vi "Climber.vi"() -> ()   [LabVIEW 2012]
uses:
  ClimberState.ctl
  <vilib>/Rock Robotics/WPI/Solenoid/WPI_SolenoidValue.ctl
  <vilib>/Rock Robotics/WPI/Relay/WPI_RelayValue.ctl
  Robot Global Data.vi
  <vilib>/Rock Robotics/WPI/Solenoid/WPI_SolenoidSetEnum.vi
  <vilib>/Rock Robotics/WPI/RobotDrive/WPI_RobotDriveGetSetRefNum.vi
panel:
  in  "Debug":bool
  in  "Step":T1
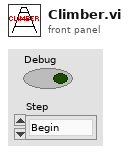
[diagram p1: front panel]
types:
  T1 = typedef "ClimberState.ctl" = enum16{"Begin", "Step 1", "Step 2", "Step 3", "Step 4", "Step 5", "Step 6", "Step 7", "Step 8", "Step 9", "Step 10", "Step 11", "Step 12", "Step 13", "Step 14", "Step 15", "Step 16", "Step 17", "Step 18", "Step 19", "Step 20", "Step 21", "Step 22", "Step 23", "End"}
  T2 = typedef "WPI_SolenoidValue.ctl" = enum16{"Off", "On", "Forward", "Reverse"}
  T3 = typedef "WPI_RelayValue.ctl" = enum16{"Off", "On", "Forward", "Reverse"}
  T4 = typedef "Level state.ctl" = enum16{"None", "Level 1", "Level 2", "Level 3"}
  T5 = typedef "WPI_SolenoidDevRef.ctl" = cluster{"DevStatus":errorcluster, "Solenoid Module":T6, "Forward Solenoid Channel":T7, "Reverse Solenoid Channel":T7}
  T6 = typedef "FPGA_TypedefSolenoidModule.ctl" = enum16{"Solenoid Module 1", "Solenoid Module 2"}
  T7 = typedef "WPI_SolenoidChannel.ctl" = enum8{"Solenoid 1", "Solenoid 2", "Solenoid 3", "Solenoid 4", "Solenoid 5", "Solenoid 6", "Solenoid 7", "Solenoid 8", "Invalid"}
  T8 = typedef "WPI_MotorControlDeviceRef.ctl" = cluster{"DeviceStatus":errorcluster, "Type":enum16{"PWM", "CAN"}, "PWM":cluster{"Digital Module":T9, "PWM Channel":T10, "DeadBand":T11}, "CAN":cluster{"Device Number":u8, "Control Mode":T12, "Semaphore":T13, "Max Vout":dbl}, "Invert":bool, "TransformRef":T14, "InvTransformRef":T14}
  T9 = typedef "FPGA_TypedefDigitalModule.ctl" = enum16{"Digital Module 1", "Digital Module 2"}
  T10 = typedef "FPGA_DIOPWMChannel.ctl" = enum8{"PWM 1", "PWM 2", "PWM 3", "PWM 4", "PWM 5", "PWM 6", "PWM 7", "PWM 8", "PWM 9", "PWM 10", "Invalid"}
  T11 = typedef "WPI_PWMDeadband.ctl" = cluster{"Name":string, "maxPositivePwm":i32, "minPositivePwm":i32, "centerPwm":i32, "maxNegativePwm":i32, "minNegativePwm":i32, "angularRange":u16}
  T12 = typedef "WPI_CANJaguar_ControlMode.ctl" = enum8{"Percent VBus", "Current", "Speed", "Position", "Voltage"}
  T13 = typedef "Semaphore RefNum" = refnum<k1>
  T14 = typedef "WPI_PWMTransform_ConPane.ctl" = refnum<vi>
  T15 = typedef "WPI_RobotDriveDevRef.ctl" = cluster{"DevStatus":errorcluster, "Motors[]":T8[], "Square Inputs":bool, "Max Output":dbl, "Isochronous":bool}
  T16 = typedef "WPI_RelayDevRef.ctl" = cluster{"DevStatus":errorcluster, "Relay Channel":T17, "Digital Module":T9, "Relay Direction":T18}
  T17 = typedef "FPGA_DIORelayChannel.ctl" = enum8{"Relay 1", "Relay 2", "Relay 3", "Relay 4", "Relay 5", "Relay 6", "Relay 7", "Relay 8", "Invalid"}
  T18 = typedef "WPI_RelayDirection.ctl" = enum16{"Both directions", "Forward only", "Reverse only"}
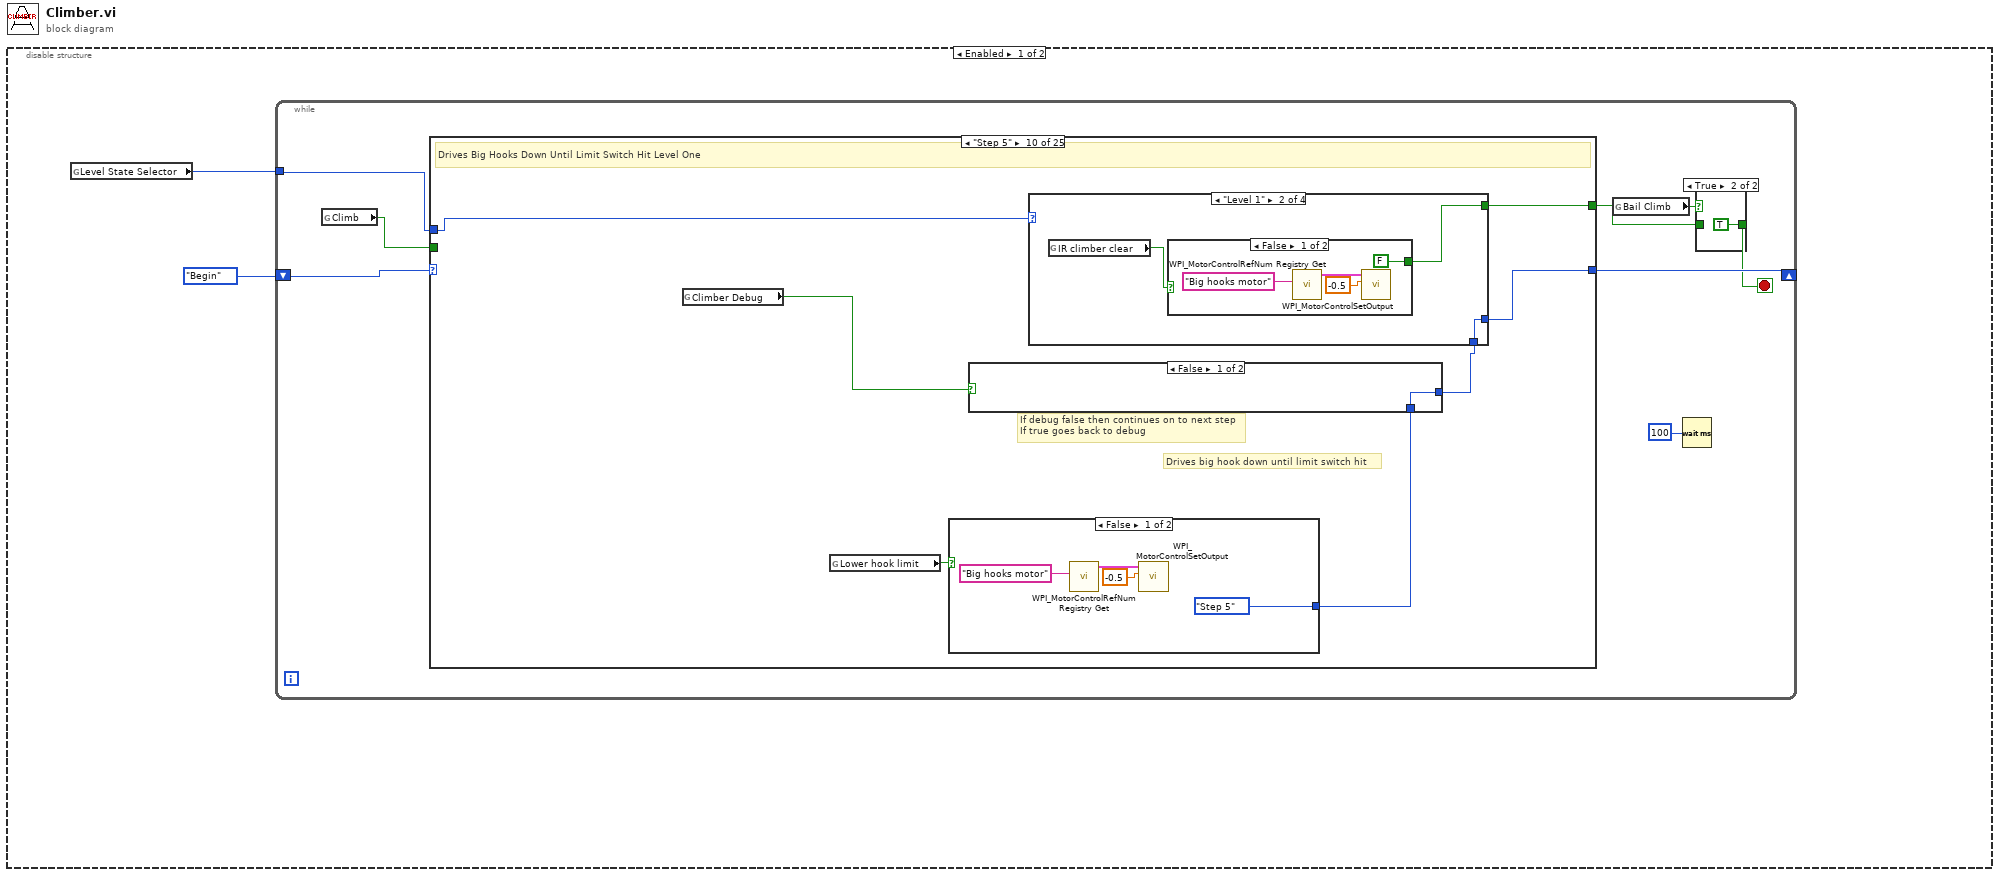
[diagram p0: block diagram]
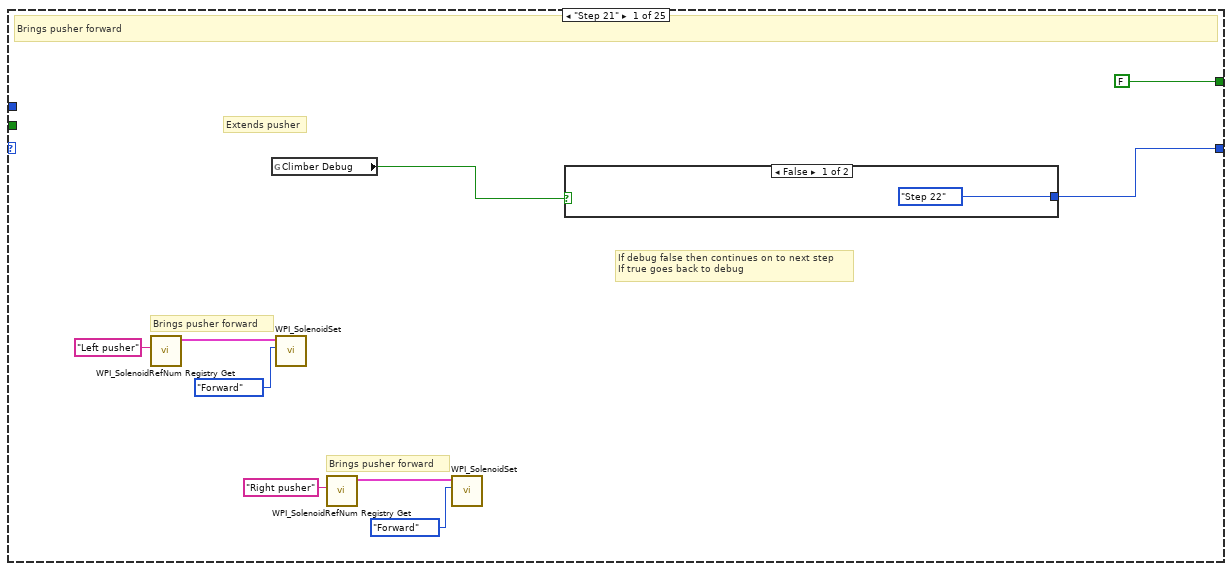
[diagram p3: hidden frame]
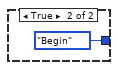
[diagram p4: hidden frame]
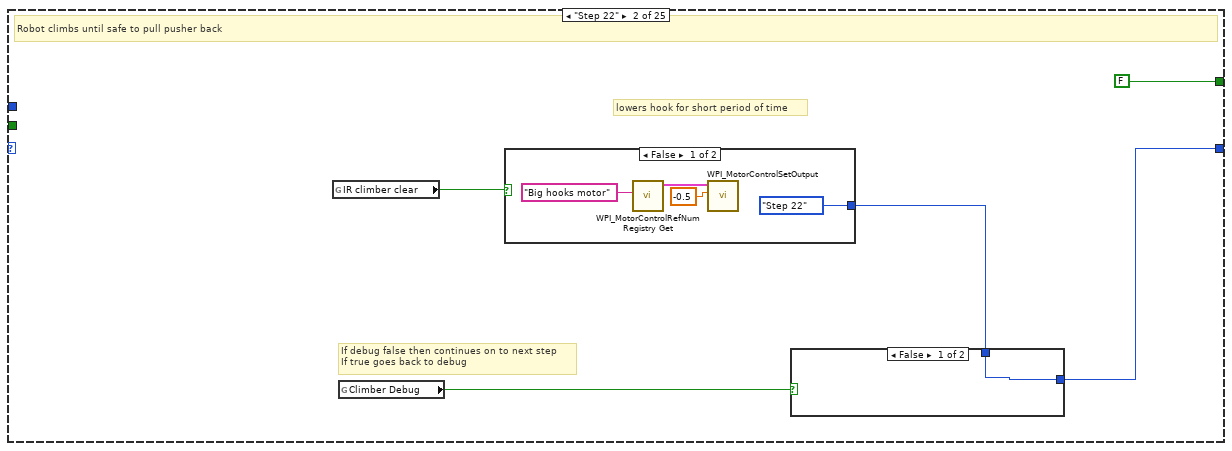
[diagram p5: hidden frame]
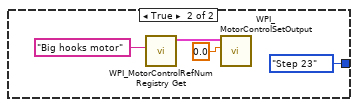
[diagram p6: hidden frame]
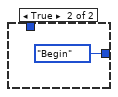
[diagram p7: hidden frame]
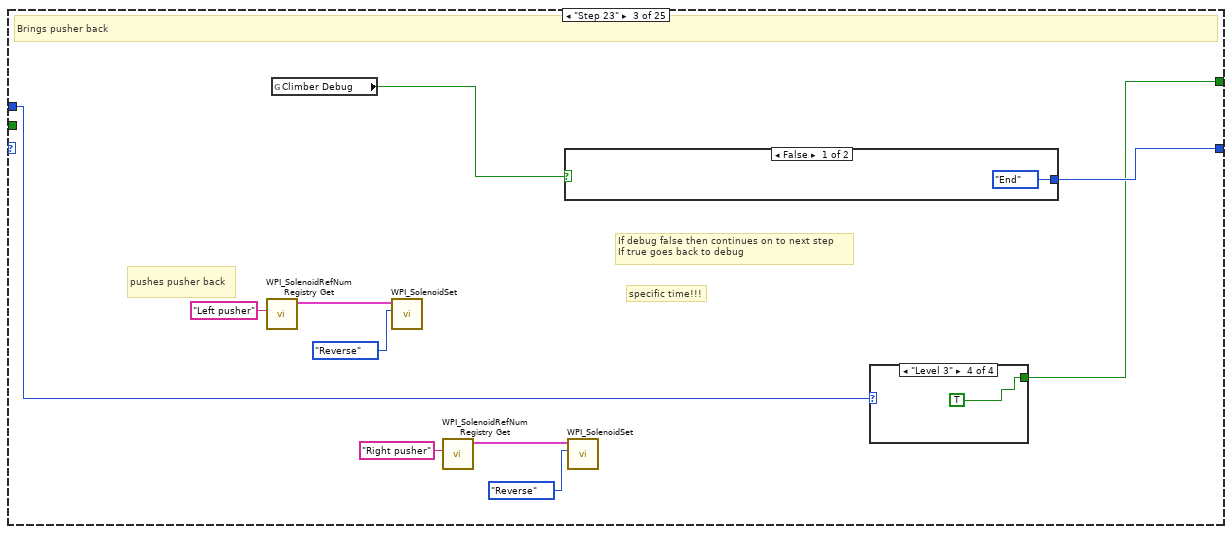
[diagram p8: hidden frame]
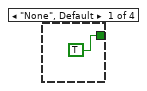
[diagram p9: hidden frame]
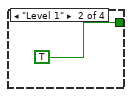
[diagram p10: hidden frame]
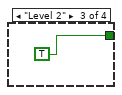
[diagram p11: hidden frame]
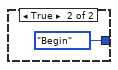
[diagram p12: hidden frame]
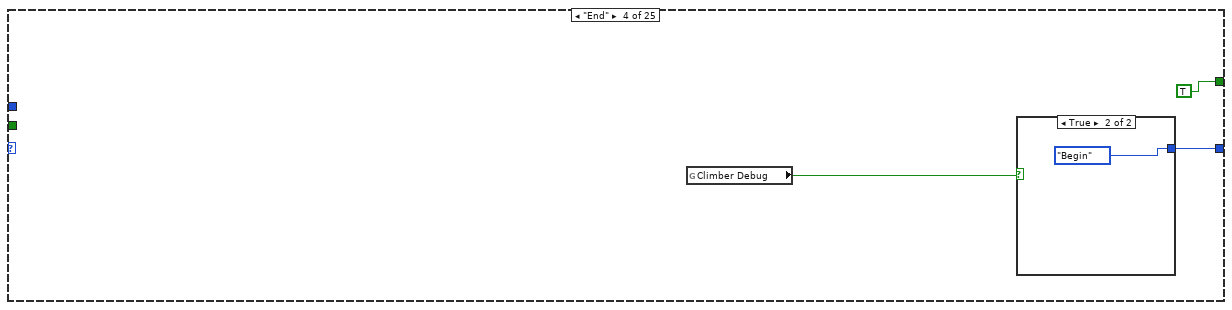
[diagram p13: hidden frame]
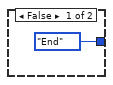
[diagram p14: hidden frame]
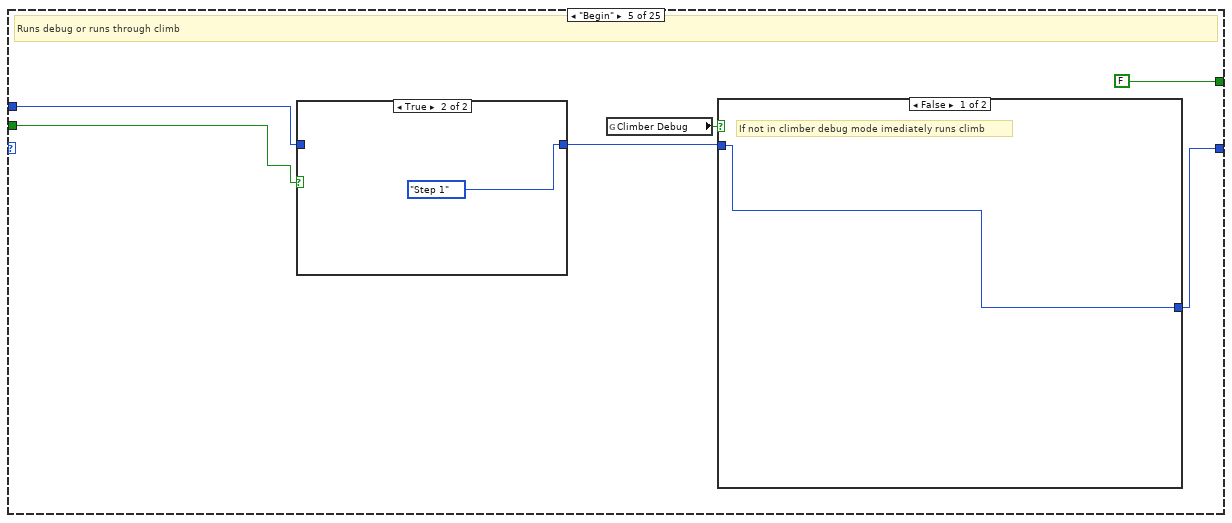
[diagram p15: hidden frame]
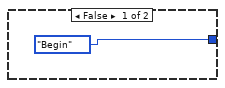
[diagram p16: hidden frame]
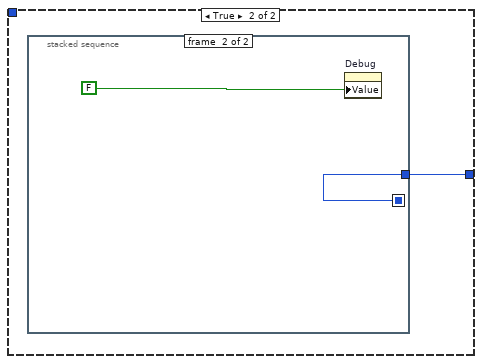
[diagram p17: hidden frame]
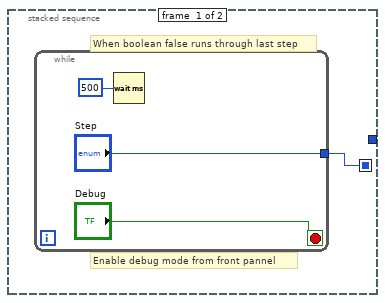
[diagram p18: hidden frame]
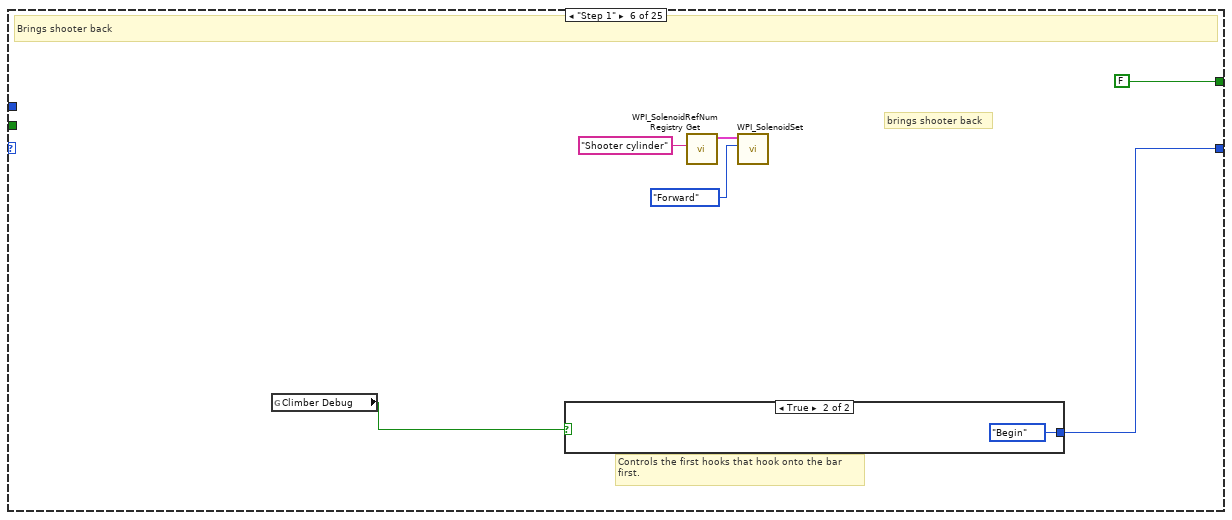
[diagram p19: hidden frame]
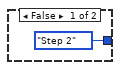
[diagram p20: hidden frame]
diagram:
  n1 = disable-structure shown="Enabled" {
    frame Enabled {
      n2 = global read "Robot Global Data.vi" "Level State Selector"() -> (w2:T4)
      n3 = while {
        shift-right: [w10] -> _
        shift-left: ClimberState."Begin" ("Enum") -> [w9]
        tunnel: w2 -> [w4]
        stop <- w8 stop-if-true
        n4 = global read "Robot Global Data.vi" "Climb"() -> (w3:bool)
        n5 = case shown="\"Step 5\"" w9 {
          tunnel: [w19 w26 w47 w56 w65 w80 w85 w104 w112 w117 w154 w160 w172 w190 w206 w217 w224 w245 w255 w271 w277 w289 w305 w312 w328] -> w10
          tunnel: [FALSE FALSE w40 TRUE FALSE FALSE FALSE FALSE FALSE w120 FALSE FALSE FALSE FALSE FALSE FALSE FALSE w238 FALSE FALSE FALSE FALSE FALSE FALSE FALSE] -> w7
          tunnel: w4 -> [_ _ w39 _ w62 _ _ _ _ w119 _ _ _ _ _ _ _ w237 _ _ _ _ _ _ _]
          tunnel: w3 -> [_ _ _ _ w60 _ _ _ _ _ _ _ _ _ _ _ _ _ _ _ _ _ _ _ _]
          frame "Step 21" {
            # "Brings pusher forward"
            # "Brings pusher forward"
            # "If debug false then continues on to next step\nIf true goes back to debug"
            # "Extends pusher"
            # "Brings pusher forward"
            n6 = call <vilib>:"WPI_SolenoidRefNum Registry Get.vi"("refnum name"="Left pusher") -> ("SolenoidDevRef"=w16:T5)  [unwired: 9 in, 1 out]
            n7 = global read "Robot Global Data.vi" "Climber Debug"() -> (w20:bool)
            n8 = call-poly <vilib>:"WPI_SolenoidSet.vi"("Value"=WPI_SolenoidValue."Forward", "SolenoidDevRef"=w16) -> ()  [unwired: 8 in, 2 out]
            n9 = call <vilib>:"WPI_SolenoidRefNum Registry Get.vi"("refnum name"="Right pusher") -> ("SolenoidDevRef"=w14:T5)  [unwired: 9 in, 1 out]
            n10 = call-poly <vilib>:"WPI_SolenoidSet.vi"("Value"=WPI_SolenoidValue."Forward", "SolenoidDevRef"=w14) -> ()  [unwired: 8 in, 2 out]
            n11 = case shown="False" w20 {
              tunnel: [ClimberState."Step 22" ("Enum") ClimberState."Begin" ("Enum")] -> w19
              frame False {
              }
              frame True {
              }
            }
          }
          frame "Step 22" {
            # "lowers hook for short period of time"
            # "If debug false then continues on to next step\nIf true goes back to debug"
            # "Robot climbs until safe to pull pusher back"
            n12 = global read "Robot Global Data.vi" "IR climber clear"() -> (w25:bool)
            n13 = global read "Robot Global Data.vi" "Climber Debug"() -> (w27:bool)
            n14 = case shown="False" w25 {
              tunnel: [ClimberState."Step 22" ("Enum") ClimberState."Step 23" ("Enum")] -> w24
              frame False {
                n15 = call <vilib>:"WPI_MotorControlRefNum Registry Get.vi"("refnum name"="Big hooks motor") -> ("MotorControlDevRef"=w30:T8)  [unwired: 9 in, 1 out]
                n16 = call <vilib>:"WPI_MotorControlSetOutput.vi"("Output"=-0.5, "MotorControlDevRef"=w30) -> ()  [unwired: 7 in, 3 out]
              }
              frame True {
                n17 = call <vilib>:"WPI_MotorControlRefNum Registry Get.vi"("refnum name"="Big hooks motor") -> ("MotorControlDevRef"=w36:T8)  [unwired: 9 in, 1 out]
                n18 = call <vilib>:"WPI_MotorControlSetOutput.vi"("Output"=0.0, "MotorControlDevRef"=w36) -> ()  [unwired: 7 in, 3 out]
              }
            }
            n19 = case shown="False" w27 {
              tunnel: [w37 ClimberState."Begin" ("Enum")] -> w26
              tunnel: w24 -> [w37 _]
              frame False {
              }
              frame True {
              }
            }
          }
          frame "Step 23" {
            # "specific time!!!"
            # "pushes pusher back"
            # "If debug false then continues on to next step\nIf true goes back to debug"
            # "Brings pusher back"
            n20 = call <vilib>:"WPI_SolenoidRefNum Registry Get.vi"("refnum name"="Left pusher") -> ("SolenoidDevRef"=w44:T5)  [unwired: 9 in, 1 out]
            n21 = global read "Robot Global Data.vi" "Climber Debug"() -> (w48:bool)
            n22 = call-poly <vilib>:"WPI_SolenoidSet.vi"("Value"=WPI_SolenoidValue."Reverse", "SolenoidDevRef"=w44) -> ()  [unwired: 8 in, 2 out]
            n23 = call <vilib>:"WPI_SolenoidRefNum Registry Get.vi"("refnum name"="Right pusher") -> ("SolenoidDevRef"=w42:T5)  [unwired: 9 in, 1 out]
            n24 = case shown="False" w48 {
              tunnel: [ClimberState."End" ("Enum") ClimberState."Begin" ("Enum")] -> w47
              frame False {
              }
              frame True {
              }
            }
            n25 = call-poly <vilib>:"WPI_SolenoidSet.vi"("Value"=WPI_SolenoidValue."Reverse", "SolenoidDevRef"=w42) -> ()  [unwired: 8 in, 2 out]
            n26 = case shown="\"Level 3\"" w39 {
              tunnel: [TRUE TRUE TRUE TRUE] -> w40
              frame "None", Default {
              }
              frame "Level 1" {
              }
              frame "Level 2" {
              }
              frame "Level 3" {
              }
            }
          }
          frame "End" {
            n27 = global read "Robot Global Data.vi" "Climber Debug"() -> (w55:bool)
            n28 = case shown="True" w55 {
              tunnel: [ClimberState."End" ("Enum") ClimberState."Begin" ("Enum")] -> w56
              frame False {
              }
              frame True {
              }
            }
          }
          frame "Begin" {
            # "Runs debug or runs through climb"
            n29 = case shown="True" w60 {
              tunnel: w62 -> [_ _]
              tunnel: [ClimberState."Begin" ("Enum") ClimberState."Step 1" ("Enum")] -> w61
              frame False {
              }
              frame True {
              }
            }
            n30 = global read "Robot Global Data.vi" "Climber Debug"() -> (w63:bool)
            n31 = case shown="False" w63 {
              tunnel: [w68 w69] -> w65
              tunnel: w61 -> [w68 _]
              frame False {
                # "If not in climber debug mode imediately runs climb"
              }
              frame True {
                n32 = stacked-sequence {
                  seq-local: [w70 _] -> [_ w75]
                  tunnel: [_ w75] -> w69
                  frame #0 {
                    # "When boolean false runs through last step"
                    # "Enable debug mode from front pannel"
                    n33 = while {
                      tunnel: ["Step"] -> w70
                      stop <- "Debug" stop-if-true
                      n34 = Wait (ms)(milliseconds to wait=u32 500) -> ()  [unwired: 1 out]
                    }
                  }
                  frame #1 {
                    n35 = property on="Debug" class="Bool (strict)"("Value"=FALSE ("Debug")) -> ()  [unwired: 2 in, 2 out]
                  }
                }
              }
            }
          }
          frame "Step 1" {
            # "brings shooter back"
            # "Controls the first hooks that hook onto the bar\nfirst."
            # "Brings shooter back"
            n36 = global read "Robot Global Data.vi" "Climber Debug"() -> (w79:bool)
            n37 = case shown="True" w79 {
              tunnel: [ClimberState."Step 2" ("Enum") ClimberState."Begin" ("Enum")] -> w80
              frame False {
              }
              frame True {
              }
            }
            n38 = call <vilib>:"WPI_SolenoidRefNum Registry Get.vi"("refnum name"="Shooter cylinder") -> ("SolenoidDevRef"=w77:T5)  [unwired: 9 in, 1 out]
            n39 = call-poly <vilib>:"WPI_SolenoidSet.vi"("Value"=WPI_SolenoidValue."Forward", "SolenoidDevRef"=w77) -> ()  [unwired: 8 in, 2 out]
          }
          frame "Step 2" {
            # "Drives hook up till limit switch hit"
            # "till hits limit switch"
            # "If debug false then continues on to next step\nIf true goes back to debug"
            # "Drives up to bar"
            # "Drives big hooks up"
            n40 = global read "Robot Global Data.vi" "Climber Debug"() -> (w87:bool)
            n41 = global read "Robot Global Data.vi" "Top hook limit"() -> (w86:bool)
            n42 = case shown="False" w86 {
              tunnel: [ClimberState."Step 2" ("Enum") ClimberState."Step 3" ("Enum")] -> w84
              frame False {
                n43 = call <vilib>:"WPI_MotorControlRefNum Registry Get.vi"("refnum name"="Big hooks motor") -> ("MotorControlDevRef"=w90:T8)  [unwired: 9 in, 1 out]
                n44 = call <vilib>:"WPI_MotorControlSetOutput.vi"("Output"=0.5, "MotorControlDevRef"=w90) -> ()  [unwired: 7 in, 3 out]
              }
              frame True {
                n45 = call <vilib>:"WPI_MotorControlRefNum Registry Get.vi"("refnum name"="Big hooks motor") -> ("MotorControlDevRef"=w96:T8)  [unwired: 9 in, 1 out]
                n46 = call <vilib>:"WPI_MotorControlSetOutput.vi"("Output"=0.0, "MotorControlDevRef"=w96) -> ()  [unwired: 7 in, 3 out]
              }
            }
            n47 = case shown="True" w87 {
              tunnel: [w97 ClimberState."Begin" ("Enum")] -> w85
              tunnel: w84 -> [w97 _]
              frame False {
              }
              frame True {
              }
            }
          }
          frame "Step 3" {
            # "Drives robot up to the tower"
            # "If debug false then continues on to next step\nIf true goes back to debug"
            # "Drives robot to tower"
            n48 = global read "Robot Global Data.vi" "Climber Debug"() -> (w105:bool)
            n49 = call <vilib>:"WPI_RobotDriveRefNum Registry Get.vi"("refnum name"="Left and Right Motors") -> ("error out"=w103:errorcluster, "RobotDriveDevRef"=w102:T15)  [unwired: 1 in, 8 out]
            n50 = call <vilib>:"WPI_RobotDriveTankDrive.vi"("error in (no error)"=w103, "Right axis value"=-0.5, "Left axis value"=-0.5, "RobotDriveDevRef"=w102) -> ()  [unwired: 5 in, 3 out]
            n51 = case shown="True" w105 {
              tunnel: [ClimberState."Step 4" ("Enum") ClimberState."Begin" ("Enum")] -> w104
              frame False {
              }
              frame True {
              }
            }
          }
          frame "Step 4" {
            # "Makes sure that Ratchet is engaged"
            # "If debug false then continues on to next step\nIf true goes back to debug"
            # "Brings Ratchet Forward to Ensure that it is Engaged"
            n52 = global read "Robot Global Data.vi" "Climber Debug"() -> (w113:bool)
            n53 = case shown="False" w113 {
              tunnel: [ClimberState."Step 5" ("Enum") ClimberState."Begin" ("Enum")] -> w112
              frame False {
              }
              frame True {
              }
            }
            n54 = call <vilib>:"WPI_SolenoidRefNum Registry Get.vi"("refnum name"="Big hooks lock") -> ("SolenoidDevRef"=w110:T5)  [unwired: 9 in, 1 out]
            n55 = call-poly <vilib>:"WPI_SolenoidSet.vi"("Value"=WPI_SolenoidValue."Forward", "SolenoidDevRef"=w110) -> ()  [unwired: 8 in, 2 out]
          }
          frame "Step 5" {
            # "Drives big hook down until limit switch hit"
            # "If debug false then continues on to next step\nIf true goes back to debug"
            # "Drives Big Hooks Down Until Limit Switch Hit Level One"
            n56 = global read "Robot Global Data.vi" "Climber Debug"() -> (w123:bool)
            n57 = global read "Robot Global Data.vi" "Lower hook limit"() -> (w122:bool)
            n58 = case shown="False" w122 {
              tunnel: [ClimberState."Step 5" ("Enum") ClimberState."Step 6" ("Enum")] -> w121
              frame False {
                n59 = call <vilib>:"WPI_MotorControlRefNum Registry Get.vi"("refnum name"="Big hooks motor") -> ("MotorControlDevRef"=w142:T8)  [unwired: 9 in, 1 out]
                n60 = call <vilib>:"WPI_MotorControlSetOutput.vi"("Output"=-0.5, "MotorControlDevRef"=w142) -> ()  [unwired: 7 in, 3 out]
              }
              frame True {
                n61 = call <vilib>:"WPI_MotorControlRefNum Registry Get.vi"("refnum name"="Big hooks motor") -> ("MotorControlDevRef"=w148:T8)  [unwired: 9 in, 1 out]
                n62 = call <vilib>:"WPI_MotorControlSetOutput.vi"("Output"=0.0, "MotorControlDevRef"=w148) -> ()  [unwired: 7 in, 3 out]
              }
            }
            n63 = case shown="False" w123 {
              tunnel: [w149 ClimberState."Begin" ("Enum")] -> w118
              tunnel: w121 -> [w149 _]
              frame False {
              }
              frame True {
              }
            }
            n64 = case shown="\"Level 1\"" w119 {
              tunnel: [TRUE w126 FALSE FALSE] -> w120
              tunnel: w118 -> [w124 w127 w137 w139]
              tunnel: [w124 w127 w137 w139] -> w117
              frame "None", Default {
              }
              frame "Level 1" {
                n65 = global read "Robot Global Data.vi" "IR climber clear"() -> (w128:bool)
                n66 = case shown="False" w128 {
                  tunnel: [FALSE TRUE] -> w126
                  frame False {
                    n67 = call <vilib>:"WPI_MotorControlRefNum Registry Get.vi"("refnum name"="Big hooks motor") -> ("MotorControlDevRef"=w132:T8)  [unwired: 9 in, 1 out]
                    n68 = call <vilib>:"WPI_MotorControlSetOutput.vi"("Output"=-0.5, "MotorControlDevRef"=w132) -> ()  [unwired: 7 in, 3 out]
                  }
                  frame True {
                    n69 = call <vilib>:"WPI_MotorControlRefNum Registry Get.vi"("refnum name"="Big hooks motor") -> ("MotorControlDevRef"=w136:T8)  [unwired: 9 in, 1 out]
                    n70 = call <vilib>:"WPI_MotorControlSetOutput.vi"("Output"=0.0, "MotorControlDevRef"=w136) -> ()  [unwired: 7 in, 3 out]
                  }
                }
              }
              frame "Level 2" {
              }
              frame "Level 3" {
              }
            }
          }
          frame "Step 6" {
            # "pushes inner hooks forward"
            # "Extends Outer Hook"
            # "If debug false then continues on to next step\nIf true goes back to debug"
            # "Brings Small Hooks Forward onto Bar"
            n71 = global read "Robot Global Data.vi" "Climber Debug"() -> (w155:bool)
            n72 = call <vilib>:"WPI_RelayRefNum Registry Get.vi"("refnum name"="Small hooks") -> ("RelayDevRef"=w153:T16)  [unwired: 9 in, 1 out]
            n73 = call <vilib>:"WPI_RelaySet.vi"("RelayValue"=WPI_RelayValue."Forward", "RelayDevRef"=w153) -> ()  [unwired: 8 in, 2 out]
            n74 = case shown="False" w155 {
              tunnel: [ClimberState."Step 7" ("Enum") ClimberState."Begin" ("Enum")] -> w154
              frame False {
              }
              frame True {
              }
            }
          }
          frame "Step 7" {
            # "Brings ratchet back then drives down for short moment"
            # "If debug false then continues on to next step\nIf true goes back to debug"
            # "Brings ratchet back and drives down"
            n75 = flat-sequence {
              frame #0 {
                n76 = call <vilib>:"WPI_SolenoidRefNum Registry Get.vi"("refnum name"="Big hooks lock") -> ("SolenoidDevRef"=w163:T5)  [unwired: 9 in, 1 out]
                n77 = call-poly <vilib>:"WPI_SolenoidSet.vi"("Value"=WPI_SolenoidValue."Reverse", "SolenoidDevRef"=w163) -> ()  [unwired: 8 in, 2 out]
              }
              frame #1 {
                n78 = call <vilib>:"WPI_MotorControlRefNum Registry Get.vi"("refnum name"="Big hooks motor") -> ("MotorControlDevRef"=w167:T8)  [unwired: 9 in, 1 out]
                n79 = call <vilib>:"WPI_MotorControlSetOutput.vi"("Output"=-0.5, "MotorControlDevRef"=w167) -> ()  [unwired: 7 in, 3 out]
              }
            }
            n80 = global read "Robot Global Data.vi" "Climber Debug"() -> (w161:bool)
            n81 = case shown="False" w161 {
              tunnel: [ClimberState."Step 8" ("Enum") ClimberState."Begin" ("Enum")] -> w160
              frame False {
              }
              frame True {
              }
            }
          }
          frame "Step 8" {
            # "till hits limit switch"
            # "If debug false then continues on to next step\nIf true goes back to debug"
            # "Extends inner hooks"
            # "Brings big hook up until limit switch hit"
            n82 = global read "Robot Global Data.vi" "Climber Debug"() -> (w173:bool)
            n83 = global read "Robot Global Data.vi" "Top hook limit"() -> (w171:bool)
            n84 = case shown="False" w171 {
              tunnel: [ClimberState."Step 8" ("Enum") ClimberState."Step 9" ("Enum")] -> w170
              frame False {
                n85 = call <vilib>:"WPI_MotorControlRefNum Registry Get.vi"("refnum name"="Big hooks motor") -> ("MotorControlDevRef"=w176:T8)  [unwired: 9 in, 1 out]
                n86 = call <vilib>:"WPI_MotorControlSetOutput.vi"("Output"=0.5, "MotorControlDevRef"=w176) -> ()  [unwired: 7 in, 3 out]
              }
              frame True {
                n87 = call <vilib>:"WPI_MotorControlRefNum Registry Get.vi"("refnum name"="Big hooks motor") -> ("MotorControlDevRef"=w182:T8)  [unwired: 9 in, 1 out]
                n88 = call <vilib>:"WPI_MotorControlSetOutput.vi"("Output"=0.0, "MotorControlDevRef"=w182) -> ()  [unwired: 7 in, 3 out]
              }
            }
            n89 = case shown="False" w173 {
              tunnel: [w183 ClimberState."Begin" ("Enum")] -> w172
              tunnel: w170 -> [w183 _]
              frame False {
              }
              frame True {
              }
            }
          }
          frame "Step 9" {
            # "Ratchet engages."
            # "If debug false then continues on to next step\nIf true goes back to debug"
            # "Brings Ratchet forward and lowers big hook"
            n90 = call <vilib>:"WPI_SolenoidRefNum Registry Get.vi"("refnum name"="Big hooks lock") -> ("SolenoidDevRef"=w188:T5)  [unwired: 9 in, 1 out]
            n91 = call-poly <vilib>:"WPI_SolenoidSet.vi"("Value"=WPI_SolenoidValue."Forward", "SolenoidDevRef"=w188) -> ()  [unwired: 8 in, 2 out]
            n92 = global read "Robot Global Data.vi" "Climber Debug"() -> (w191:bool)
            n93 = global read "Robot Global Data.vi" "Big Hooks on Bar"() -> (w186:bool)
            n94 = case shown="False" w186 {
              tunnel: [ClimberState."Step 9" ("Enum") ClimberState."Step 10" ("Enum")] -> w185
              frame False {
                # "Lowers the big hooks"
                n95 = call <vilib>:"WPI_MotorControlRefNum Registry Get.vi"("refnum name"="Big hooks motor") -> ("MotorControlDevRef"=w196:T8)  [unwired: 9 in, 1 out]
                n96 = call <vilib>:"WPI_MotorControlSetOutput.vi"("Output"=-0.5, "MotorControlDevRef"=w196) -> ()  [unwired: 7 in, 3 out]
              }
              frame True {
                n97 = call <vilib>:"WPI_MotorControlRefNum Registry Get.vi"("refnum name"="Big hooks motor") -> ("MotorControlDevRef"=w199:T8)  [unwired: 9 in, 1 out]
                n98 = call <vilib>:"WPI_MotorControlSetOutput.vi"("Output"=0.0, "MotorControlDevRef"=w199) -> ()  [unwired: 7 in, 3 out]
              }
            }
            n99 = case shown="False" w191 {
              tunnel: [w201 ClimberState."Begin" ("Enum")] -> w190
              tunnel: w185 -> [w201 _]
              frame False {
              }
              frame True {
              }
            }
          }
          frame "Step 10" {
            # "Bring small inner hooks back"
            # "If debug false then continues on to next step\nIf true goes back to debug"
            # "Brings small inner hooks back"
            n100 = global read "Robot Global Data.vi" "Climber Debug"() -> (w207:bool)
            n101 = call <vilib>:"WPI_RelayRefNum Registry Get.vi"("refnum name"="Small hooks") -> ("RelayDevRef"=w205:T16)  [unwired: 9 in, 1 out]
            n102 = case shown="False" w207 {
              tunnel: [ClimberState."Step 11" ("Enum") ClimberState."Begin" ("Enum")] -> w206
              frame False {
              }
              frame True {
              }
            }
            n103 = call <vilib>:"WPI_RelaySet.vi"("RelayValue"=WPI_RelayValue."Reverse", "RelayDevRef"=w205) -> ()  [unwired: 8 in, 2 out]
          }
          frame "Step 11" {
            # "Brings pusher forward"
            # "If debug false then continues on to next step\nIf true goes back to debug"
            # "Brings pusher forward"
            # "Extends inner hooks"
            # "Pusher pushes robot forward"
            n104 = global read "Robot Global Data.vi" "Climber Debug"() -> (w218:bool)
            n105 = call <vilib>:"WPI_SolenoidRefNum Registry Get.vi"("refnum name"="Left pusher") -> ("SolenoidDevRef"=w214:T5)  [unwired: 9 in, 1 out]
            n106 = call-poly <vilib>:"WPI_SolenoidSet.vi"("Value"=WPI_SolenoidValue."Forward", "SolenoidDevRef"=w214) -> ()  [unwired: 8 in, 2 out]
            n107 = call <vilib>:"WPI_SolenoidRefNum Registry Get.vi"("refnum name"="Right pusher") -> ("SolenoidDevRef"=w212:T5)  [unwired: 9 in, 1 out]
            n108 = case shown="False" w218 {
              tunnel: [ClimberState."Step 12" ("Enum") ClimberState."Begin" ("Enum")] -> w217
              frame False {
              }
              frame True {
              }
            }
            n109 = call-poly <vilib>:"WPI_SolenoidSet.vi"("Value"=WPI_SolenoidValue."Forward", "SolenoidDevRef"=w212) -> ()  [unwired: 8 in, 2 out]
          }
          frame "Step 12" {
            # "lowers big hook for short period of time"
            # "If debug false then continues on to next step\nIf true goes back to debug"
            # "Extends Outer Hook"
            # "Robot climbs until safe to pull pusher back"
            n110 = global read "Robot Global Data.vi" "Climber Debug"() -> (w225:bool)
            n111 = global read "Robot Global Data.vi" "IR climber clear"() -> (w223:bool)
            n112 = case shown="False" w223 {
              tunnel: [ClimberState."Step 12" ("Enum") ClimberState."Step 13" ("Enum")] -> w222
              frame False {
                n113 = call <vilib>:"WPI_MotorControlRefNum Registry Get.vi"("refnum name"="Big hooks motor") -> ("MotorControlDevRef"=w228:T8)  [unwired: 9 in, 1 out]
                n114 = call <vilib>:"WPI_MotorControlSetOutput.vi"("Output"=-0.5, "MotorControlDevRef"=w228) -> ()  [unwired: 7 in, 3 out]
              }
              frame True {
                n115 = call <vilib>:"WPI_MotorControlRefNum Registry Get.vi"("refnum name"="Big hooks motor") -> ("MotorControlDevRef"=w234:T8)  [unwired: 9 in, 1 out]
                n116 = call <vilib>:"WPI_MotorControlSetOutput.vi"("Output"=0.0, "MotorControlDevRef"=w234) -> ()  [unwired: 7 in, 3 out]
              }
            }
            n117 = case shown="False" w225 {
              tunnel: [w235 ClimberState."Begin" ("Enum")] -> w224
              tunnel: w222 -> [w235 _]
              frame False {
              }
              frame True {
              }
            }
          }
          frame "Step 13" {
            # "find specific time"
            # "Brings pusher back"
            # "Brings pusher back"
            # "brings pusher cyliner back"
            # "If debug false then continues on to next step\nIf true goes back to debug"
            # "Pusher reverses Level two"
            n118 = call <vilib>:"WPI_SolenoidRefNum Registry Get.vi"("refnum name"="Left pusher") -> ("SolenoidDevRef"=w242:T5)  [unwired: 9 in, 1 out]
            n119 = call-poly <vilib>:"WPI_SolenoidSet.vi"("Value"=WPI_SolenoidValue."Reverse", "SolenoidDevRef"=w242) -> ()  [unwired: 8 in, 2 out]
            n120 = call <vilib>:"WPI_SolenoidRefNum Registry Get.vi"("refnum name"="Right pusher") -> ("SolenoidDevRef"=w240:T5)  [unwired: 9 in, 1 out]
            n121 = global read "Robot Global Data.vi" "Climber Debug"() -> (w246:bool)
            n122 = call-poly <vilib>:"WPI_SolenoidSet.vi"("Value"=WPI_SolenoidValue."Reverse", "SolenoidDevRef"=w240) -> ()  [unwired: 8 in, 2 out]
            n123 = case shown="False" w246 {
              tunnel: [ClimberState."Step 14" ("Enum") ClimberState."Begin" ("Enum")] -> w245
              frame False {
              }
              frame True {
              }
            }
            n124 = case shown="\"Level 2\"" w237 {
              tunnel: [TRUE TRUE TRUE FALSE] -> w238
              frame "None", Default {
              }
              frame "Level 1" {
              }
              frame "Level 2" {
              }
              frame "Level 3" {
              }
            }
          }
          frame "Step 14" {
            # "till hits limit switch"
            # "lowers big hook"
            # "Robot climbs rest of way up"
            n125 = global read "Robot Global Data.vi" "Climber Debug"() -> (w256:bool)
            n126 = global read "Robot Global Data.vi" "Lower hook limit"() -> (w254:bool)
            n127 = case shown="False" w254 {
              tunnel: [ClimberState."Step 14" ("Enum") ClimberState."Step 15" ("Enum")] -> w253
              frame False {
                n128 = call <vilib>:"WPI_MotorControlRefNum Registry Get.vi"("refnum name"="Big hooks motor") -> ("MotorControlDevRef"=w259:T8)  [unwired: 9 in, 1 out]
                n129 = call <vilib>:"WPI_MotorControlSetOutput.vi"("Output"=-0.5, "MotorControlDevRef"=w259) -> ()  [unwired: 7 in, 3 out]
              }
              frame True {
                n130 = call <vilib>:"WPI_MotorControlRefNum Registry Get.vi"("refnum name"="Big hooks motor") -> ("MotorControlDevRef"=w265:T8)  [unwired: 9 in, 1 out]
                n131 = call <vilib>:"WPI_MotorControlSetOutput.vi"("Output"=0.0, "MotorControlDevRef"=w265) -> ()  [unwired: 7 in, 3 out]
              }
            }
            n132 = case shown="False" w256 {
              tunnel: [w266 ClimberState."Begin" ("Enum")] -> w255
              tunnel: w253 -> [w266 _]
              frame False {
              }
              frame True {
              }
            }
          }
          frame "Step 15" {
            # "brings small inner hooks forward"
            # "If debug false then continues on to next step\nIf true goes back to debug"
            # "Brings small hooks forward till they are on bar"
            n133 = global read "Robot Global Data.vi" "Climber Debug"() -> (w272:bool)
            n134 = call <vilib>:"WPI_RelayRefNum Registry Get.vi"("refnum name"="Small hooks") -> ("RelayDevRef"=w270:T16)  [unwired: 9 in, 1 out]
            n135 = case shown="True" w272 {
              tunnel: [ClimberState."Step 16" ("Enum") ClimberState."Begin" ("Enum")] -> w271
              frame False {
              }
              frame True {
              }
            }
            n136 = call <vilib>:"WPI_RelaySet.vi"("RelayValue"=WPI_RelayValue."Forward", "RelayDevRef"=w270) -> ()  [unwired: 8 in, 2 out]
          }
          frame "Step 16" {
            # "brings ratchet back and then brings big hook down"
            # "If debug false then continues on to next step\nIf true goes back to debug"
            # "Brings ratchet back and drives down"
            n137 = flat-sequence {
              frame #0 {
                n138 = call <vilib>:"WPI_SolenoidRefNum Registry Get.vi"("refnum name"="Big hooks lock") -> ("SolenoidDevRef"=w280:T5)  [unwired: 9 in, 1 out]
                n139 = call-poly <vilib>:"WPI_SolenoidSet.vi"("Value"=WPI_SolenoidValue."Reverse", "SolenoidDevRef"=w280) -> ()  [unwired: 8 in, 2 out]
              }
              frame #1 {
                n140 = call <vilib>:"WPI_MotorControlRefNum Registry Get.vi"("refnum name"="Big hooks motor") -> ("MotorControlDevRef"=w284:T8)  [unwired: 9 in, 1 out]
                n141 = call <vilib>:"WPI_MotorControlSetOutput.vi"("Output"=-0.5, "MotorControlDevRef"=w284) -> ()  [unwired: 7 in, 3 out]
              }
            }
            n142 = global read "Robot Global Data.vi" "Climber Debug"() -> (w278:bool)
            n143 = case shown="False" w278 {
              tunnel: [ClimberState."Step 17" ("Enum") ClimberState."Begin" ("Enum")] -> w277
              frame False {
              }
              frame True {
              }
            }
          }
          frame "Step 17" {
            # "brings big hook up"
            # "till hits limit switch"
            # "Brings big hook up until limit switch activated"
            n144 = global read "Robot Global Data.vi" "Top hook limit"() -> (w288:bool)
            n145 = global read "Robot Global Data.vi" "Climber Debug"() -> (w290:bool)
            n146 = case shown="False" w288 {
              tunnel: [ClimberState."Step 17" ("Enum") ClimberState."Step 18" ("Enum")] -> w287
              frame False {
                n147 = call <vilib>:"WPI_MotorControlRefNum Registry Get.vi"("refnum name"="Big hooks motor") -> ("MotorControlDevRef"=w293:T8)  [unwired: 9 in, 1 out]
                n148 = call <vilib>:"WPI_MotorControlSetOutput.vi"("Output"=0.5, "MotorControlDevRef"=w293) -> ()  [unwired: 7 in, 3 out]
              }
              frame True {
                n149 = call <vilib>:"WPI_MotorControlRefNum Registry Get.vi"("refnum name"="Big hooks motor") -> ("MotorControlDevRef"=w299:T8)  [unwired: 9 in, 1 out]
                n150 = call <vilib>:"WPI_MotorControlSetOutput.vi"("Output"=0.0, "MotorControlDevRef"=w299) -> ()  [unwired: 7 in, 3 out]
              }
            }
            n151 = case shown="False" w290 {
              tunnel: [w300 ClimberState."Begin" ("Enum")] -> w289
              tunnel: w287 -> [w300 _]
              frame False {
              }
              frame True {
              }
            }
          }
          frame "Step 18" {
            # "engage ratchet"
            # "If debug false then continues on to next step\nIf true goes back to debug"
            # "Extends inner hooks"
            # "Brings ratchet forward"
            n152 = global read "Robot Global Data.vi" "Climber Debug"() -> (w306:bool)
            n153 = call <vilib>:"WPI_SolenoidRefNum Registry Get.vi"("refnum name"="Big hooks lock") -> ("SolenoidDevRef"=w303:T5)  [unwired: 9 in, 1 out]
            n154 = call-poly <vilib>:"WPI_SolenoidSet.vi"("Value"=WPI_SolenoidValue."Forward", "SolenoidDevRef"=w303) -> ()  [unwired: 8 in, 2 out]
            n155 = case shown="False" w306 {
              tunnel: [ClimberState."Step 19" ("Enum") ClimberState."Begin" ("Enum")] -> w305
              frame False {
              }
              frame True {
              }
            }
          }
          frame "Step 19" {
            # "If debug false then continues on to next step\nIf true goes back to debug"
            # "Brings big hooks down until they are on bar"
            n156 = global read "Robot Global Data.vi" "Big Hooks on Bar"() -> (w311:bool)
            n157 = case shown="False" w311 {
              tunnel: [ClimberState."Step 19" ("Enum") ClimberState."Step 20" ("Enum")] -> w310
              frame False {
                # "Lowers the big hook until proximity hit"
                n158 = call <vilib>:"WPI_MotorControlRefNum Registry Get.vi"("refnum name"="Big hooks motor") -> ("MotorControlDevRef"=w318:T8)  [unwired: 9 in, 1 out]
                n159 = call <vilib>:"WPI_MotorControlSetOutput.vi"("Output"=-0.5, "MotorControlDevRef"=w318) -> ()  [unwired: 7 in, 3 out]
              }
              frame True {
                n160 = call <vilib>:"WPI_MotorControlRefNum Registry Get.vi"("refnum name"="Big hooks motor") -> ("MotorControlDevRef"=w321:T8)  [unwired: 9 in, 1 out]
                n161 = call <vilib>:"WPI_MotorControlSetOutput.vi"("Output"=0.0, "MotorControlDevRef"=w321) -> ()  [unwired: 7 in, 3 out]
              }
            }
            n162 = global read "Robot Global Data.vi" "Climber Debug"() -> (w313:bool)
            n163 = case shown="False" w313 {
              tunnel: [w323 ClimberState."Begin" ("Enum")] -> w312
              tunnel: w310 -> [w323 _]
              frame False {
              }
              frame True {
              }
            }
          }
          frame "Step 20" {
            # "disengage small hooks"
            # "If debug false then continues on to next step\nIf true goes back to debug"
            # "Brings small hooks back"
            n164 = global read "Robot Global Data.vi" "Climber Debug"() -> (w329:bool)
            n165 = call <vilib>:"WPI_RelayRefNum Registry Get.vi"("refnum name"="Small hooks") -> ("RelayDevRef"=w327:T16)  [unwired: 9 in, 1 out]
            n166 = case shown="False" w329 {
              tunnel: [ClimberState."Step 21" ("Enum") ClimberState."Begin" ("Enum")] -> w328
              frame False {
              }
              frame True {
              }
            }
            n167 = call <vilib>:"WPI_RelaySet.vi"("RelayValue"=WPI_RelayValue."Reverse", "RelayDevRef"=w327) -> ()  [unwired: 8 in, 2 out]
          }
        }
        n168 = global read "Robot Global Data.vi" "Bail Climb"() -> (w6:bool)
        n169 = Wait (ms)(milliseconds to wait=u32 100) -> ()  [unwired: 1 out]
        n170 = case shown="True" w6 {
          tunnel: [w11 TRUE] -> w8
          tunnel: w7 -> [w11 _]
          frame False {
          }
          frame True {
          }
        }
      }
    }
    frame Disabled {
    }
  }
